vi "Serialize Core.vi"(8 "error in (no error)":errorcluster, 11 "Serializable Message in":refnum<class "Update Number Msg.lvclass">) -> (0 "error out":errorcluster, 2 "Serialized Message":string)   [LabVIEW 2020, in "Chat Window.lvlib" / "Update Number Msg.lvclass"]
uses:
  Update Number Msg.lvclass
  Update Number Msg.lvclass/Update Number Msg.ctl
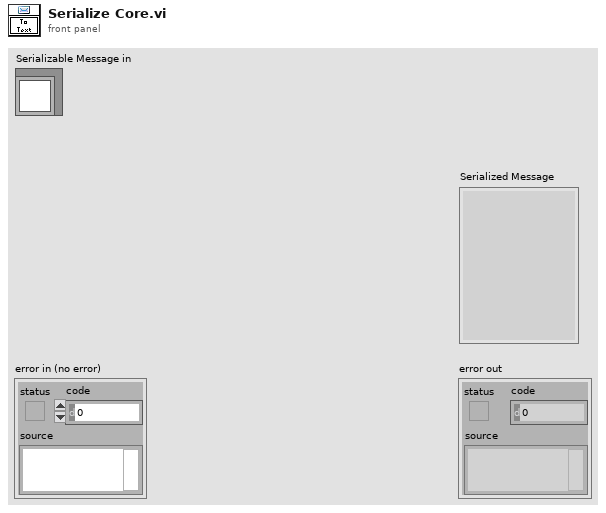
[diagram p1: front panel]
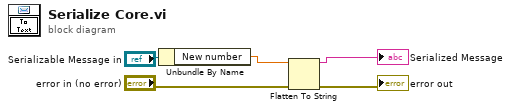
[diagram p0: block diagram]
diagram:
  n1 = Unbundle By Name("Serializable Message in") -> ("New number"=w3:dbl)
  n2 = Flatten To String(anything=w3, error in (no error)="error in (no error)") -> (data string=→"Serialized Message":string, error out=→"error out":errorcluster)  [unwired: 2 in, 1 out]
